vi "Query All Banks Cycles.vi"(8 "error in":errorcluster, 11 "ProXR_IO in":refnum<class "ProXR_IO.lvclass">) -> (0 "error out":errorcluster, 2 "Query All Banks":u8[](array[numeric]), 3 "ProXR_IO out":refnum<class "ProXR_IO.lvclass">)   [LabVIEW 2019, in "ProXR_IO.lvlib" / "ProXR_IO.lvclass"]
uses:
  ProXR_IO.lvclass
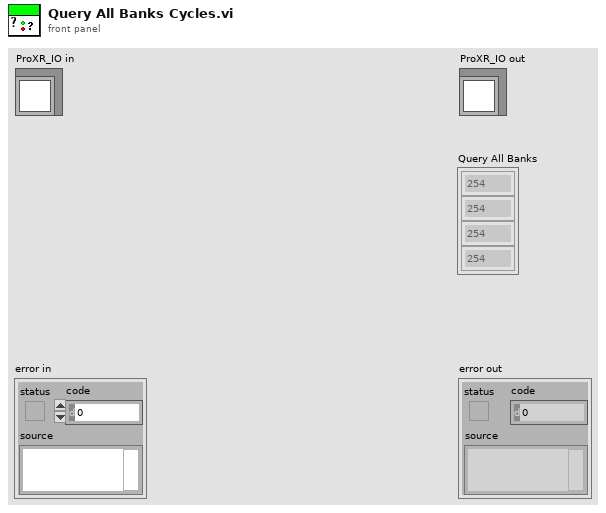
[diagram p1: front panel]
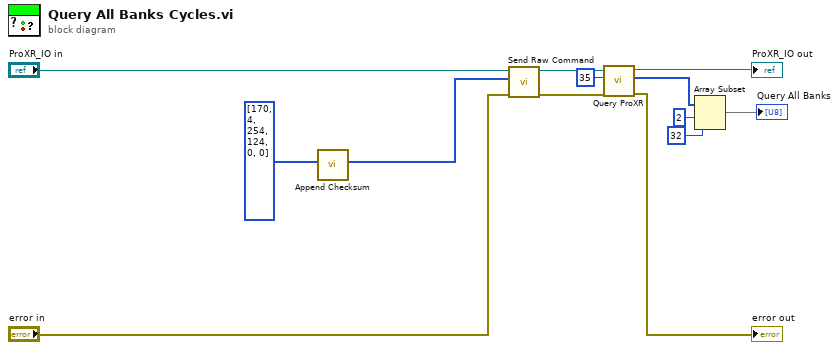
[diagram p0: block diagram]
diagram:
  n1 = call "Append Checksum.vi"("Message"=u8[] [170, 4, 254, 124, 0, 0]) -> ("Message w cksum"=w12:u8[])  [unwired: 9 in, 1 out]
  n2 = call "Send Raw Command.vi"("error in"="error in", "Raw Command"=w12, "ProXR_IO in"="ProXR_IO in") -> ("error out"=w10:errorcluster, "ProXR_IO out"=w9:refnum<class "ProXR_IO.lvclass">)  [unwired: 7 in]
  n3 = call "Query ProXR.vi"("error in"=w10, "Bytes to Read"=u32 35, "ProXR_IO in"=w9) -> ("error out"=→"error out":errorcluster, "Response"=w3:u8[], "ProXR_IO out"=→"ProXR_IO out":refnum<class "ProXR_IO.lvclass">)  [unwired: 6 in]
  n4 = Array Subset(array=w3, index=2, length=32) -> (→"Query All Banks":u8[])
